vi "Binary Search on One Hot Encoded Number (U64).vi"(7 "One Hot Encoded Number":u64 format="%064b") -> (8 "Binary Number":u8)   [LabVIEW 2010]
doc: "This VI gives the index the index of first one from LSB. It assumes that the number is one hot encoded.\nInother words it converts one hot encoded number to Binary Number"
panel:
  out "a[5]":bool
  out "a[3]":bool
  out "a[4]":bool
  out "Binary Array":bool[](array[boolean])
  out "a[0]":bool
  out "a[1]":bool
  out "a[2]":bool
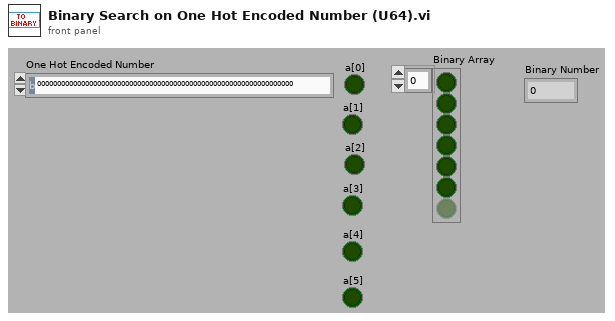
[diagram p1: front panel]
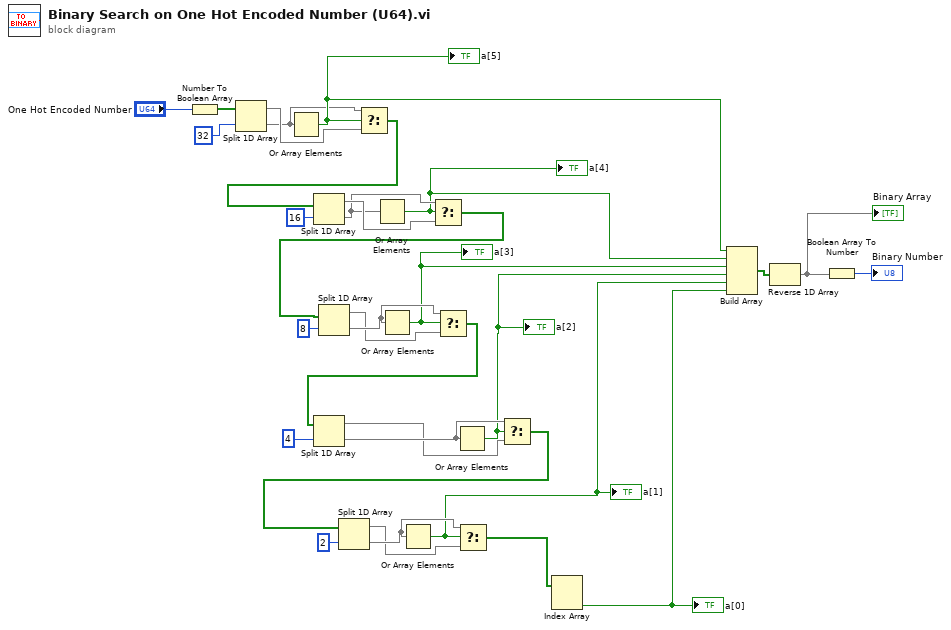
[diagram p0: block diagram]
diagram:
  n1 = Number To Boolean Array(number="One Hot Encoded Number") -> (Boolean array=w6:bool[])
  n2 = Split 1D Array(array=w6, index=32) -> (first subarray=w2:bool[], second subarray=w1:bool[])
  n3 = Or Array Elements(Boolean array=w1) -> (logical OR=w3:bool)
  "a[5]" <- w3
  n4 = Select(t=w1, s=w3, f=w2) -> (s? t:f=w4:bool[])
  n5 = Split 1D Array(array=w4, index=16) -> (first subarray=w18:bool[], second subarray=w17:bool[])
  n6 = Or Array Elements(Boolean array=w17) -> (logical OR=w10:bool)
  "a[4]" <- w10
  n7 = Select(t=w17, s=w10, f=w18) -> (s? t:f=w12:bool[])
  n8 = Split 1D Array(array=w12, index=8) -> (first subarray=w13:bool[], second subarray=w14:bool[])
  n9 = Or Array Elements(Boolean array=w14) -> (logical OR=w8:bool)
  "a[3]" <- w8
  n10 = Select(t=w14, s=w8, f=w13) -> (s? t:f=w11:bool[])
  n11 = Split 1D Array(array=w11, index=4) -> (first subarray=w29:bool[], second subarray=w30:bool[])
  n12 = Or Array Elements(Boolean array=w30) -> (logical OR=w9:bool)
  "a[2]" <- w9
  n13 = Select(t=w30, s=w9, f=w29) -> (s? t:f=w28:bool[])
  n14 = Split 1D Array(array=w28, index=2) -> (first subarray=w25:bool[], second subarray=w26:bool[])
  n15 = Or Array Elements(Boolean array=w26) -> (logical OR=w24:bool)
  "a[1]" <- w24
  n16 = Select(t=w26, s=w24, f=w25) -> (s? t:f=w20:bool[])
  n17 = Index Array(array=w20) -> (element #2=w19:bool)  [unwired: 2 in, 1 out]
  "a[0]" <- w19
  n18 = Build Array(w3, w10, w8, w9, w24, w19) -> (w23:bool[])
  n19 = Reverse 1D Array(array=w23) -> (reversed array=w21:bool[])
  "Binary Array" <- w21
  n20 = Boolean Array To Number(Boolean array=w21) -> (number=→"Binary Number":u8)
